vi "Get Frame Documentation.vi"(5 "Remove EOLs? (TRUE)":bool=TRUE, 7 "Event Structure (F: Case Structure)":bool, 8 "error in (no error)":errorcluster, 9 "State Name":string, 10 "Category (Optional)":string, 11 "JKI SM in":refnum<class "JKI SM.lvclass">) -> (0 "error out":errorcluster, 2 "Documentation":string, 3 "JKI SM out":refnum<class "JKI SM.lvclass">)   [LabVIEW 2013, in "JKI State Machine API.lvlib" / "JKI SM.lvclass"]
uses:
  JKI SM.lvclass
  JKI SM.lvclass/JKI SM.ctl
  <userlib>/_OpenG.lib/string/string.llb/Convert EOLs (String)__ogtk.vi
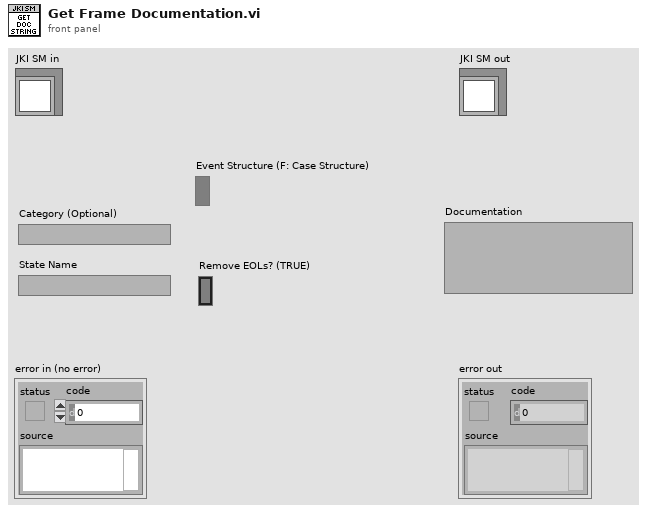
[diagram p1: front panel]
types:
  T1 = typedef "LVBoundsTypeDef.ctl" = cluster{"Width":u32, "Height":u32}
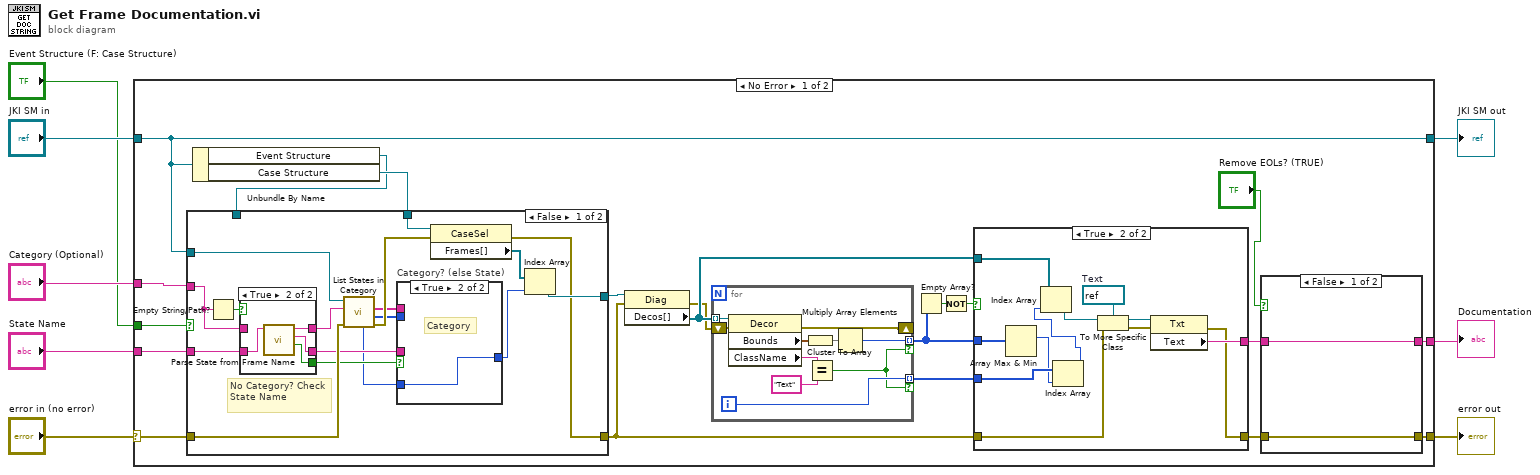
[diagram p0: block diagram]
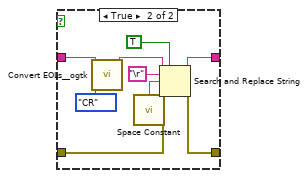
[diagram p2: hidden frame]
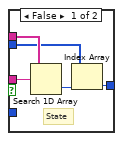
[diagram p4: hidden frame]
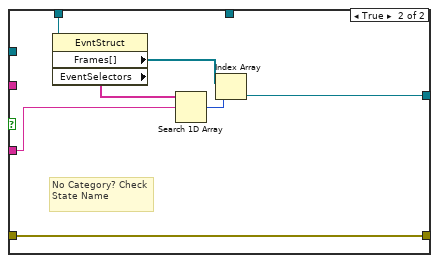
[diagram p6: hidden frame]
diagram:
  n1 = case shown="No Error" "error in (no error)" {
    selector: "error in (no error)" -> [w24 w100]
    tunnel: [w11 w100] -> w7
    tunnel: [w25 w99] -> w5
    tunnel: "JKI SM in" -> [w25 w99]
    tunnel: "State Name" -> [w26 _]
    tunnel: "Category (Optional)" -> [w27 _]
    tunnel: "Event Structure (F: Case Structure)" -> [w23 _]
    tunnel: [w10 _] -> w1
    frame No Error {
      n2 = Unbundle By Name(w25) -> ("Event Structure"=w22:refnum<vi>, "Case Structure"=w28:refnum<vi>)
      n3 = case shown="False" w23 {
        tunnel: [w67 w97] -> w17
        tunnel: w28 -> [w72 _]
        tunnel: w27 -> [w78 _]
        tunnel: w26 -> [w77 w98]
        tunnel: w25 -> [w76 _]
        tunnel: w24 -> [w75 w97]
        tunnel: w22 -> [_ w96]
        tunnel: [w69 w92] -> w21
        frame False {
          # "No Category? Check State Name"
          n4 = Empty String/Path?(string/path=w78) -> (empty?=w79:bool)
          n5 = case shown="True" w79 {
            tunnel: w77 -> [w86 w91]
            tunnel: [w87 w90] -> w74
            tunnel: w78 -> [w87 _]
            tunnel: [w86 w89] -> w73
            tunnel: [_ w88] -> w64
            frame False {
            }
            frame True {
              n6 = call "Parse State from Frame Name.vi"("Frame or State Name"=w91) -> ("is a Category Frame?"=w88:bool, "State Name"=w89:string, "Category Name"=w90:string)  [unwired: 6 in, 2 out]
            }
          }
          n7 = call "List States in Category.vi"("error in (no error)"=w75, "Category"=w74, "JKI SM in"=w76) -> ("error out"=w68:errorcluster, "State Frame Indices"=w65:i32[], "States"=w66:string[], "Category Frame Index"=w63:i32)  [unwired: 4 in, 1 out]
          n8 = case "Category? (else State)" shown="True" w64 {
            tunnel: w73 -> [w84 _]
            tunnel: [w83 w85] -> w71
            tunnel: w66 -> [w82 _]
            tunnel: w65 -> [w81 _]
            tunnel: w63 -> [_ w85]
            frame False {
              # "State"
              n9 = Search 1D Array(1D array=w82, element=w84) -> (index of element=w80:i32)  [unwired: 1 in]
              n10 = Index Array(array=w81, index=w80) -> (element=w83:i32)
            }
            frame True {
              # "Category"
            }
          }
          n11 = property class="CaseSel"(reference=w72, error in=w68) -> (error out=w67:errorcluster, "Frames[]"=w70:refnum<vi>[])  [unwired: 1 out]
          n12 = Index Array(array=w70, index=w71) -> (element=w69:refnum<vi>)
        }
        frame True {
          # "No Category? Check State Name"
          n13 = property class="EvntStruct"(reference=w96) -> ("Frames[]"=w93:refnum<vi>[], "EventSelectors"=w95:string[])  [unwired: 1 in, 2 out]
          n14 = Search 1D Array(1D array=w95, element=w98) -> (index of element=w94:i32)  [unwired: 1 in]
          n15 = Index Array(array=w93, index=w94) -> (element=w92:refnum<vi>)
        }
      }
      n16 = property class="Diag"(reference=w21, error in=w17) -> (error out=w19:errorcluster, "Decos[]"=w20:refnum<vi>[])  [unwired: 1 out]
      n17 = for {
        tunnel: w20 -> [w62] mode=indexing
        tunnel: [w59] -> w16 mode=indexing if=w53
        shift-right: [w57] -> _
        shift-left: w19 -> [w58]
        tunnel: [w54] -> w18 mode=indexing if=w53
        i -> [w54]
        n18 = property class="Decor"(reference=w62, error in=w58) -> (error out=w57:errorcluster, "Bounds"=w61:T1, "ClassName"=w56:string)  [unwired: 1 out]
        n19 = Cluster To Array(cluster=w61) -> (array=w60:u32[])
        n20 = Equal?(x=w56, y="Text" ("Class Name")) -> (x = y?=w53:bool)
        n21 = Multiply Array Elements(1:w60) -> (0:w59:u32)
      }
      n22 = Empty Array?(array=w16) -> (empty?=w15:bool)
      n23 = Not(x=w15) -> (.not. x?=w14:bool)
      n24 = case shown="True" w14 {
        tunnel: w20 -> [_ w52]
        tunnel: w18 -> [_ w50]
        tunnel: w17 -> [w40 w44]
        tunnel: [_ w43] -> w13
        tunnel: [w40 w42] -> w12
        tunnel: w16 -> [_ w41]
        frame False {
        }
        frame True {
          w46 = refnum<vi> refnum  # Text
          n25 = Array Max & Min(array=w41) -> (max index (indices)=w49:i32)  [unwired: 3 out]
          n26 = Index Array(array=w50, index=w49) -> (element=w48:i32)
          n27 = Index Array(array=w52, index=w48) -> (element=w51:refnum<vi>)
          n28 = To More Specific Class(target class=w46, reference=w51, error in=w44) -> (specific class reference=w47:refnum<vi>, error out=w45:errorcluster)
          n29 = property class="Txt"(reference=w47, error in=w45) -> (error out=w42:errorcluster, "Text"=w43:string)  [unwired: 1 out]
        }
      }
      n30 = case shown="False" "Remove EOLs? (TRUE)" {
        tunnel: w13 -> [w30 w39]
        tunnel: w12 -> [w29 w33]
        tunnel: [w29 w32] -> w11
        tunnel: [w30 w31] -> w10
        frame False {
        }
        frame True {
          n31 = call-poly <userlib>:"Convert EOLs__ogtk.vi"("Convert to:"=enum16{"CR", "LF", "CRLF"}."CR", "String in"=w39) -> ("String out"=w38:string)  [unwired: 9 in]
          n32 = call <vilib>:"Space Constant.vi"() -> ("String"=w34:string)
          n33 = Search and Replace String(replace all?=TRUE ("replace all? (F)"), input string=w38, search string="\r", replace string=w34, error in=w33) -> (result string=w31:string, error out=w32:errorcluster)  [unwired: 3 in, 2 out]
        }
      }
    }
    frame Error {
    }
  }
  "error out" <- w7
  "JKI SM out" <- w5
  "Documentation" <- w1
